vi "From 2D Float Tree Data.vi"(11 "Tree Data":refnum<class "Tree Data.lvclass">) -> (2 "2D Flt":dbl[][](array[numeric]))   [LabVIEW 2017, in "Tree API.lvlib" / "2D Flt.lvclass"]
doc: "Extract a 2D Float value from Tree Data type."
uses:
  2D Flt.lvclass
  Tree Data/Tree Data.lvclass
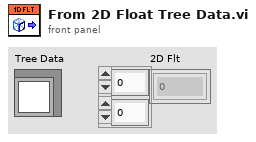
[diagram p1: front panel]
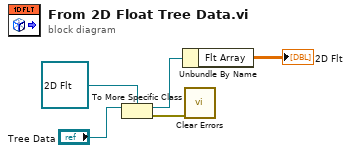
[diagram p0: block diagram]
diagram:
  n1 = To More Specific Class(target class=refnum<class "2D Flt.lvclass"> refnum ("Tree API.lvlib:2D Flt.lvclass"), reference="Tree Data") -> (specific class reference=w4:refnum<class "2D Flt.lvclass">, error out=w3:errorcluster)  [unwired: 1 in]
  n2 = Unbundle By Name(w4) -> ("Flt Array"=→"2D Flt":dbl[][])
  n3 = call <vilib>:"Clear Errors.vi"("error in (no error)"=w3) -> ()  [unwired: 5 in, 2 out]
